vi "Wash Step Control_AE.vi"(7 "Step Actions":T3, 8 "error in (no error)":errorcluster, 9 "Car Position Slider":T1 scale=0.0..4.0, 11 "Wash Options":T4) -> (0 "error out":errorcluster, 1 "Done with Washing?":bool, 2 "Current Wash Step":T5, 3 "Car Wash Indicators":T2)   [LabVIEW 2010]
doc: "Manages the state control of the wash steps.\nAllows setting of the initial steps and then sequencing to the next one"
uses:
  Controls/Current Wash Step ENUM_TDef.ctl
  Controls/Wash Options Cluster_TDef.ctl
  Controls/Step Control Methods ENUM_TDef.ctl
  Controls/Car Wash Indicators Cluster_TDef.ctl
  Controls/Car Position Slider_TDef.ctl
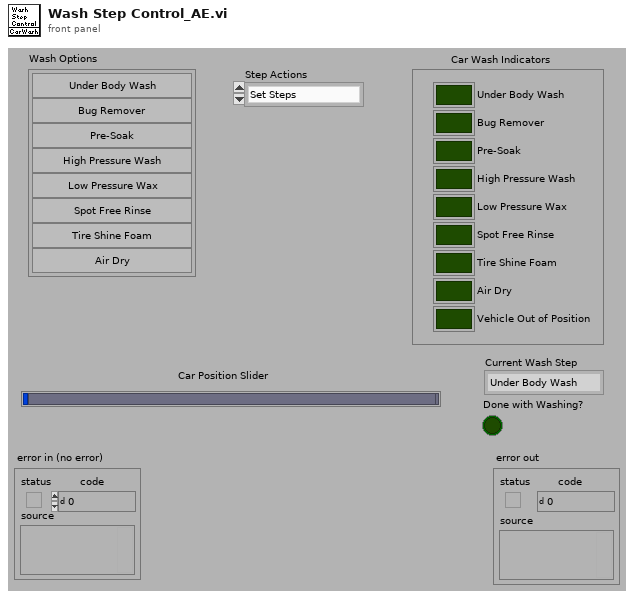
[diagram p1: front panel]
types:
  T1 = typedef "Car Position Slider_TDef.ctl" = u32
  T2 = typedef "Car Wash Indicators Cluster_TDef.ctl" = cluster{"Under Body Wash":bool, "Bug Remover":bool, "Pre-Soak":bool, "High Pressure Wash":bool, "Low Pressure Wax":bool, "Spot Free Rinse":bool, "Tire Shine Foam":bool, "Air Dry":bool, "Vehicle Out of Position":bool}
  T3 = typedef "Step Control Methods ENUM_TDef.ctl" = enum16{"Set Steps", "Get Current", "Goto Next Step"}
  T4 = typedef "Wash Options Cluster_TDef.ctl" = cluster{"Under Body Wash":bool, "Bug Remover":bool, "Pre-Soak":bool, "High Pressure Wash":bool, "Low Pressure Wax":bool, "Spot Free Rinse":bool, "Tire Shine Foam":bool, "Air Dry":bool}
  T5 = typedef "Current Wash Step ENUM_TDef.ctl" = enum16{"Under Body Wash", "Bug Remover", "Pre-Soak", "High Pressure Wash", "Low Pressure Wax", "Spot Free Rinse", "Tire Shine Foam", "Air Dry"}
  T6 = cluster{"Car Wash Indicators[0]":bool, "Car Wash Indicators[1]":bool, "Car Wash Indicators[2]":bool, "Car Wash Indicators[3]":bool, "Car Wash Indicators[4]":bool, "Car Wash Indicators[5]":bool, "Car Wash Indicators[6]":bool, "Car Wash Indicators[7]":bool, "Car Wash Indicators[8]":bool}
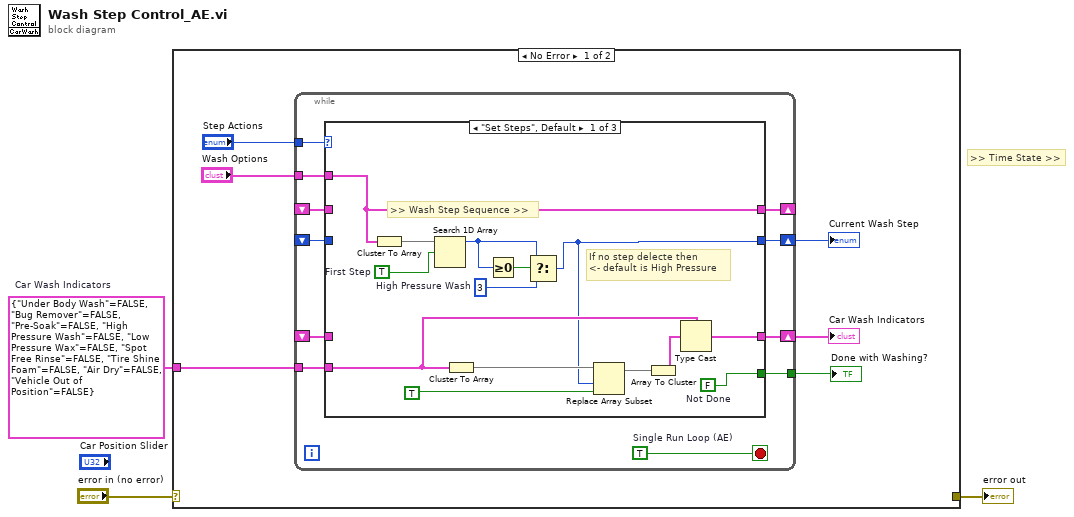
[diagram p0: block diagram]
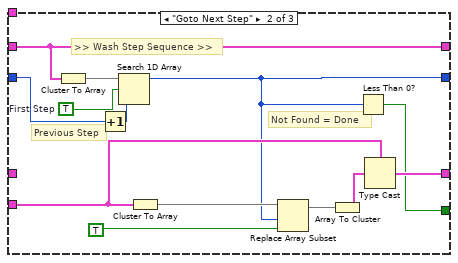
[diagram p2: hidden frame]
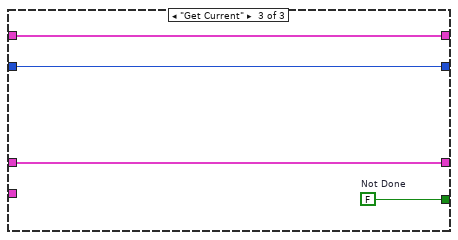
[diagram p3: hidden frame]
diagram:
  w1 = T2 {"Under Body Wash"=FALSE, "Bug Remover"=FALSE, "Pre-Soak"=FALSE, "High Pressure Wash"=FALSE, "Low Pressure Wax"=FALSE, "Spot Free Rinse"=FALSE, "Tire Shine Foam"=FALSE, "Air Dry"=FALSE, "Vehicle Out of Position"=FALSE}  # Car Wash Indicators
  # ">> Time State >>"
  n1 = case shown="No Error" "error in (no error)" {
    selector: "error in (no error)" -> [_ w52]
    tunnel: [_ w52] -> w2
    tunnel: w1 -> [w6 _]
    frame No Error {
      n2 = while {
        tunnel: "Step Actions" -> [w19]
        shift-right: [w17] -> _
        shift-left: _ -> [w16]
        tunnel: "Wash Options" -> [w18]
        shift-right: [w15] -> w7
        shift-left: _ -> [w14]
        shift-right: [w12] -> w5
        shift-left: _ -> [w11]
        tunnel: w6 -> [w13]
        tunnel: [w10] -> w4
        stop <- w20 stop-if-true
        w20 = TRUE  # Single Run Loop (AE)
        n3 = case shown="\"Set Steps\", Default" w19 {
          tunnel: w18 -> [w34 _ _]
          tunnel: [w34 w39 w49] -> w17
          tunnel: w16 -> [_ w39 w49]
          tunnel: [w22 w36 w50] -> w15
          tunnel: w14 -> [_ w38 w50]
          tunnel: w13 -> [w26 w40 _]
          tunnel: [w27 w41 w51] -> w12
          tunnel: w11 -> [_ _ w51]
          tunnel: [w25 w37 w48] -> w10
          frame "Set Steps", Default {
            w21 = 3  # High Pressure Wash
            w25 = FALSE  # Not Done
            w32 = TRUE  # First Step
            # "If no step delecte then\n<- default is High Pressure"
            # ">> Wash Step Sequence >>"
            n4 = Cluster To Array(cluster=w34) -> (array=w33:bool[])
            n5 = Search 1D Array(1D array=w33, element=w32) -> (index of element=w23:i32)  [unwired: 1 in]
            n6 = Cluster To Array(cluster=w26) -> (array=w31:bool[])
            n7 = Greater Or Equal To 0?(x=w23) -> (x >= 0?=w24:bool)
            n8 = Select(t=w23, s=w24, f=w21) -> (s? t:f=w22:i32)
            n9 = Replace Array Subset(array=w31, new element=TRUE, index=w22) -> (w29:bool[])
            n10 = Array To Cluster(array=w29) -> (cluster=w28:T6)
            n11 = Type Cast(type=w26, x=w28) -> (*(type *) &x=w27:T2)
          }
          frame "Goto Next Step" {
            w46 = TRUE  # First Step
            # "Not Found = Done"
            # "Previous Step"
            # ">> Wash Step Sequence >>"
            n12 = Cluster To Array(cluster=w39) -> (array=w47:bool[])
            n13 = Increment(x=w38) -> (x+1=w35:i32)
            n14 = Search 1D Array(1D array=w47, element=w46, start index (0)=w35) -> (index of element=w36:i32)
            n15 = Cluster To Array(cluster=w40) -> (array=w45:bool[])
            n16 = Replace Array Subset(array=w45, new element=TRUE, index=w36) -> (w43:bool[])
            n17 = Array To Cluster(array=w43) -> (cluster=w42:T6)
            n18 = Less Than 0?(x=w36) -> (x < 0?=w37:bool)
            n19 = Type Cast(type=w40, x=w42) -> (*(type *) &x=w41:T2)
          }
          frame "Get Current" {
            w48 = FALSE  # Not Done
          }
        }
      }
      "Current Wash Step" <- w7
      "Car Wash Indicators" <- w5
      "Done with Washing?" <- w4
    }
    frame Error {
    }
  }
  "error out" <- w2
